vi "ROSErrorCheck.vi"(2 "message":string, 3 "ROS in":T1) -> (1 "ROS out":T1)   [LabVIEW 2013]
uses:
  SubVIs/_ROSControl.ctl
  SubVIs/_ROSDirection.ctl
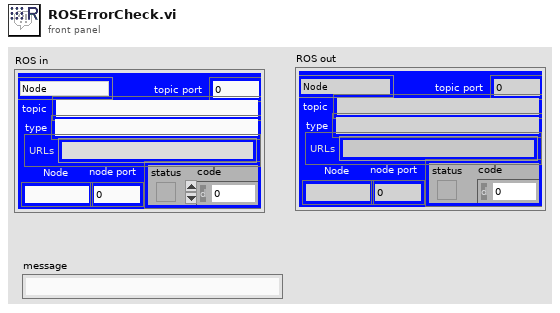
[diagram p1: front panel]
types:
  T1 = typedef "_ROSControl.ctl" = cluster{"topic port":u16, "Node":string, "topic":string, "type":string, "node port":u32, "error ":errorcluster, "Direction":T2, "APIs":string[]}
  T2 = typedef "_ROSDirection.ctl" = enum16{"Node", "Publisher", "Subscriber", "Service Client"}
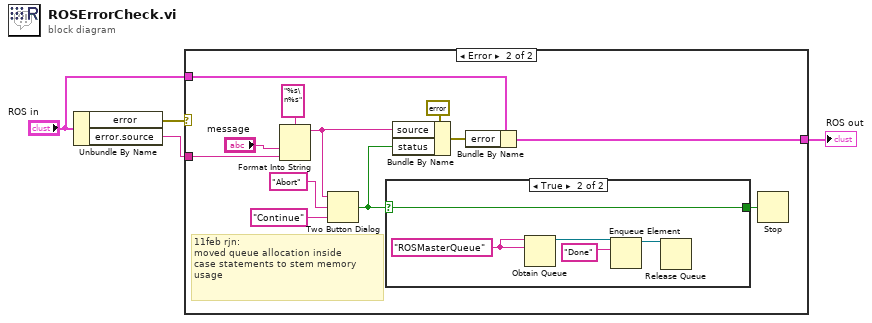
[diagram p0: block diagram]
diagram:
  n1 = Unbundle By Name("ROS in") -> ("error"=w2:errorcluster, "error.source"=w1:string)
  n2 = case shown="Error" w2 {
    tunnel: [w5 w17] -> w4
    tunnel: "ROS in" -> [w5 w16]
    tunnel: w1 -> [_ w9]
    frame No Error {
    }
    frame Error {
      # "11feb rjn:\nmoved queue allocation inside \ncase statements to stem memory usage"
      n3 = Format Into String(format string="%s\n%s", "message", w9) -> (resulting string=w8:string)  [unwired: 2 in, 1 out]
      n4 = Two Button Dialog(message=w8, 1:"Continue" ("F button name (\"Cancel\")"), 2:"Abort" ("T button name (\"OK\")")) -> (T button?=w7:bool)
      n5 = case shown="True" w7 {
        selector: w7 -> [w18 w21]
        tunnel: [w18 w21] -> w6
        frame False {
        }
        frame True {
          w20 = "ROSMasterQueue" ("name (unnamed)")
          n6 = Obtain Queue(name (unnamed)=w20, element data type=w20) -> (queue out=w19:refnum<queue>)  [unwired: 3 in, 2 out]
          n7 = Enqueue Element(queue=w19, element="Done") -> (queue out=w22:refnum<queue>)  [unwired: 2 in, 2 out]
          n8 = Release Queue(queue=w22) -> ()  [unwired: 2 in, 3 out]
        }
      }
      n9 = Bundle By Name(cluster=errorcluster {"status"=TRUE, "code"=0, "source"="Bad Topic"} ("error"), "source"=w8, "status"=w7) -> (w14:errorcluster)
      n10 = Bundle By Name(cluster=w16, "error"=w14) -> (w17:T1)
      n11 = Stop(stop? (T)=w6) -> ()
    }
  }
  "ROS out" <- w4
